vi "CRC 16.vi"(1 "input HEX string":string) -> (0 "output HEX string":string)   [LabVIEW 2023]
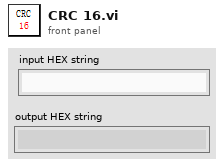
[diagram p1: front panel]
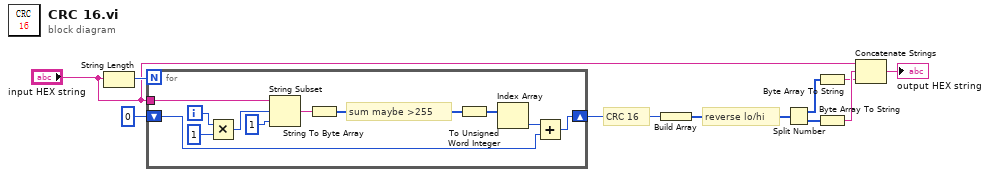
[diagram p0: block diagram]
diagram:
  # "CRC 16"
  # "reverse lo/hi"
  n1 = String Length(string="input HEX string") -> (length=w10:i32)
  n2 = for {
    N: w10 -> [_]
    tunnel: "input HEX string" -> [w13]
    shift-right: [w15] -> w8
    shift-left: u8 0 -> [w17]
    i -> [w18]
    # "sum maybe >255"
    n3 = Multiply(x=w18, y=1) -> (x*y=w21:i32)
    n4 = String Subset(string=w13, offset (0)=w21, length (rest)=1 ("length (rest)")) -> (substring=w16:string)
    n5 = String To Byte Array(string=w16) -> (unsigned byte array=w12:u8[])
    n6 = To Unsigned Word Integer(number=w12) -> (unsigned 16bit integer=w11:u16[])
    n7 = Index Array(array=w11) -> (element=w14:u16)  [unwired: 1 in]
    n8 = Add(x=w14, y=w17) -> (x+y=w15:u16)
  }
  n9 = Build Array(w8) -> (w7:u16[])
  n10 = Split Number(x=w7) -> (hi(x)=w4:u8[], lo(x)=w5:u8[])
  n11 = Byte Array To String(unsigned byte array=w4) -> (string=w2:string)
  n12 = Byte Array To String(unsigned byte array=w5) -> (string=w3:string)
  n13 = Concatenate Strings("input HEX string", w3, w2) -> (→"output HEX string":string)
